vi "Email_or_SMS.vi"(0 "Email address":string[](array[string])) -> (2 "Email":string[](array[string]))   [LabVIEW 2020]
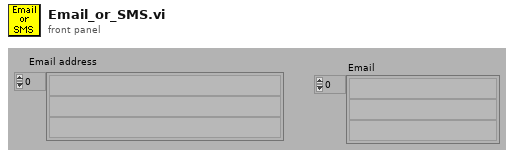
[diagram p1: front panel]
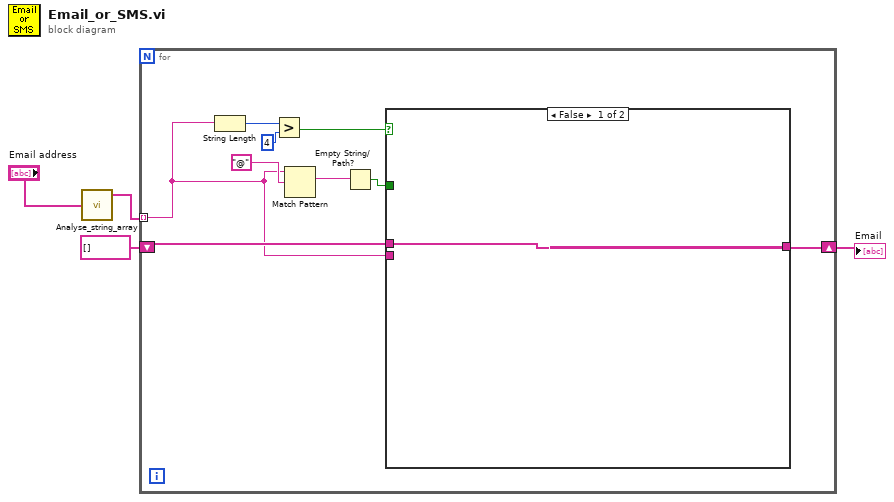
[diagram p0: block diagram]
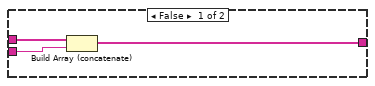
[diagram p3: hidden frame]
diagram:
  n1 = call "Analyse_string_array.vi"("String array"="Email address") -> ("Unique strings"=w4:string[])  [unwired: 2 out]
  n2 = for {
    tunnel: w4 -> [w6] mode=indexing
    shift-right: [w11] -> w3
    shift-left: string[] [] -> [w12]
    n3 = String Length(string=w6) -> (length=w10:i32)
    n4 = Greater?(x=w10, y=4) -> (0:w8:bool)
    n5 = Match Pattern(string=w6, regular expression="@") -> (match substring=w5:string)  [unwired: 4 out]
    n6 = Empty String/Path?(string/path=w5) -> (empty?=w13:bool)
    n7 = case shown="False" w8 {
      tunnel: w13 -> [_ w18]
      tunnel: w12 -> [w14 w17]
      tunnel: [w14 w16] -> w11
      tunnel: w6 -> [_ w15]
      frame False {
      }
      frame True {
        n8 = case shown="True" w18 {
          tunnel: w17 -> [w21 w22]
          tunnel: w15 -> [w20 _]
          tunnel: [w19 w22] -> w16
          frame False {
            n9 = Build Array (concatenate)(w21, w20) -> (w19:string[])
          }
          frame True {
          }
        }
      }
    }
  }
  "Email" <- w3
